vi "Substract Images.vi"() -> ()   [LabVIEW 2015]
uses:
  <vilib>/vision/NI_Vision_Development_Module.lvlib
panel:
  out "error out 3":errorcluster
  out "error out 2":errorcluster
  out "error out":errorcluster
  out "Image Dst Out":T1(plugin-control)
  in  "Image Path 2":path caption="Image Path"
  in  "Image Path":path
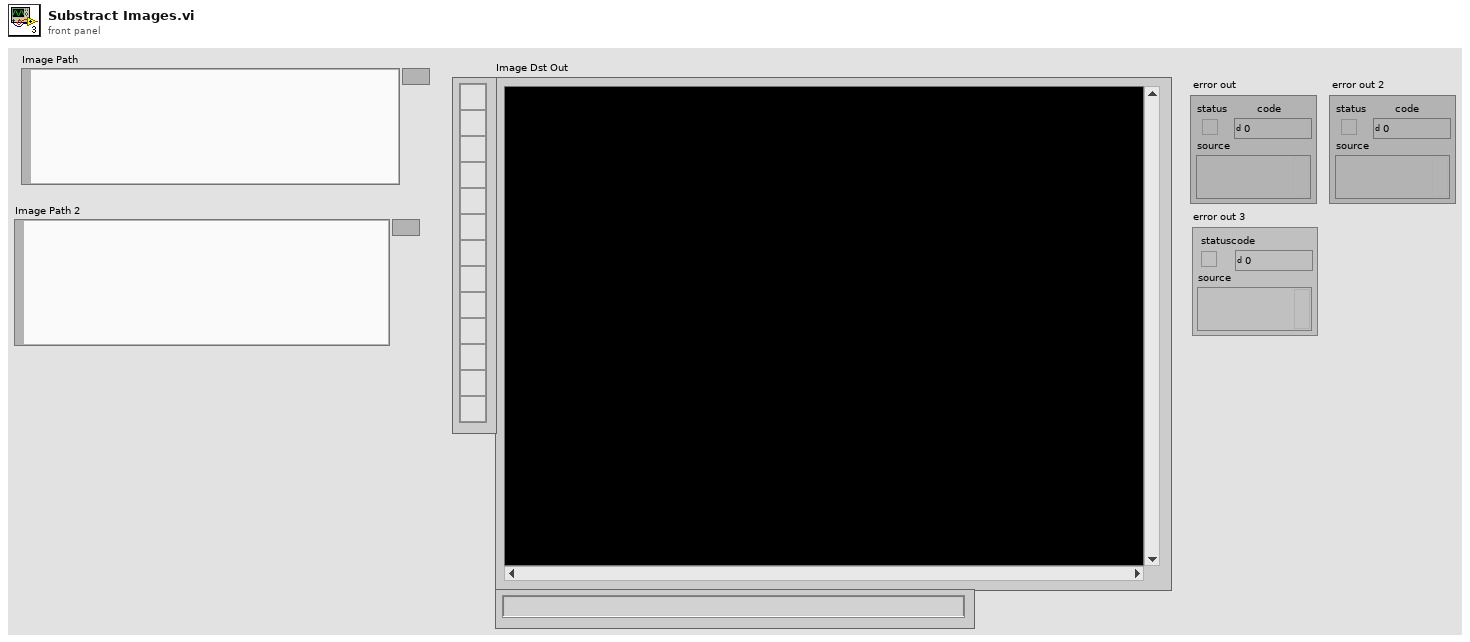
[diagram p1: front panel]
types:
  T1 = typedef "IMAQ Image.ctl" = refnum<image>
  T2 = typedef "Image Type" = u32
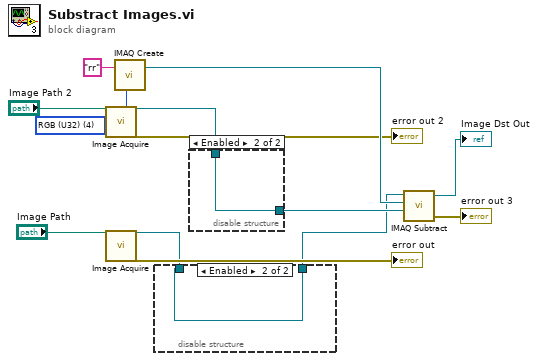
[diagram p0: block diagram]
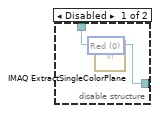
[diagram p2: hidden frame]
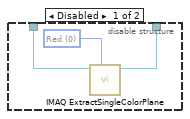
[diagram p3: hidden frame]
diagram:
  w1 = T2 4 items=["Grayscale (U8)", "Grayscale (I16)", "Grayscale (SGL)", "Complex (CSG)", "RGB (U32)", "HSL (U32)", "RGB (U64)", "Grayscale (U16)"] ("Image Type")
  n1 = call "Image Acquire.vi"("Image Path"="Image Path 2") -> ("Image Out"=w2:T1, "error out"=→"error out 2":errorcluster)  [unwired: 25 in]
  n2 = call "Image Acquire.vi"("Image Path"="Image Path") -> ("Image Out"=w4:T1, "error out"=→"error out":errorcluster)  [unwired: 25 in]
  n3 = call "IMAQ Create"("Image Name"="rr", "Image Type"=w1) -> ("New Image"=w10:T1)  [unwired: 3 in, 1 out]
  n4 = disable-structure shown="Enabled" {
    disable-tunnel: w4 -> [w15 w17]
    disable-tunnel: [w14 w17] -> w3
    frame Disabled {
      w16 = 0 items=["Red", "Green", "Blue", "Hue", "Saturation", "Luminance", "Value", "Intensity"] ("Color Plane")
      n5 = call "IMAQ ExtractSingleColorPlane"("Color Plane"=w16, "Image Src"=w15) -> ("Image Dst Out"=w14:T1)  [unwired: 8 in, 1 out]
    }
    frame Enabled {
    }
  }
  n6 = disable-structure shown="Enabled" {
    disable-tunnel: [w19 w21] -> w5
    disable-tunnel: w2 -> [w18 w21]
    frame Disabled {
      w20 = 0 items=["Red", "Green", "Blue", "Hue", "Saturation", "Luminance", "Value", "Intensity"] ("Color Plane")
      n7 = call "IMAQ ExtractSingleColorPlane"("Color Plane"=w20, "Image Src"=w18) -> ("Image Dst Out"=w19:T1)  [unwired: 8 in, 1 out]
    }
    frame Enabled {
    }
  }
  n8 = call "IMAQ Subtract"("Image Src A"=w3, "Image Dst"=w10, "Image Src B"=w5) -> ("Image Dst Out"=→"Image Dst Out":T1, "error out"=→"error out 3":errorcluster)  [unwired: 4 in]
